vi "Generation.vi"(8 "error in":errorcluster, 10 "queue in":refnum<queue>, 11 "User Event in":refnum<user-event>) -> (0 "error out":errorcluster)   [LabVIEW 2016]
uses:
  DataEvent.ctl
  DataEvent/EventType.ctl
  Generation/GenerationAndAcquisitionEnum.ctl
  FGV/GetSetEnum.ctl
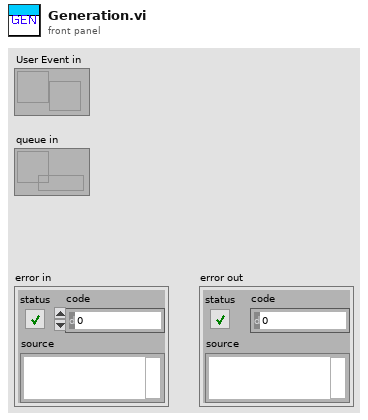
[diagram p1: front panel]
types:
  T1 = typedef "GenerationAndAcquisitionEnum.ctl" = enum16{"Idle", "Initialization", "GenerationAndPlayback", "End", "Error"}
  T2 = typedef "GetSetEnum.ctl" = enum16{"Init", "Get", "Set"}
  T3 = typedef "DataEvent.ctl" = cluster{"event type":T4, "data":variant}
  T4 = typedef "EventType.ctl" = enum16{"spectrum", "time", "exit"}
  T5 = typedef "ASIOData.ctl" = cluster{"Buffer Config":cluster{"# buffers":i32, "Buffer size":i32, "unit (ms)":enum16{"time (ms)", "Samples"}}, "Format (44kHz, 16Bit, stereo)":cluster{"Rate":i32, "Bits":i32, "Channels":u32}, "Play":bool, "Exit":bool}
  T6 = cluster{"# buffers":i32, "Buffer size":i32, "unit (ms)":enum16{"time (ms)", "Samples"}}
  T7 = typedef "SoundHandle.ctl" = cluster{"DeviceID":u16, "Samples/buf":u32, "Sampl rate":u32, "Bits/sample":u16, "Channels":u8, "Opened":bool}
  T8 = typedef "FMInfo.ctl" = cluster{"buffer size":i32, "bits":i32, "CarrierInfo":cluster{"frequency":dbl, "amplitude":dbl, "sample rate":i32, "waveform type":T9}, "ModulatorInfo":cluster{"frequency":dbl, "amplitude":dbl, "sample rate":i32, "waveform type":T9}, "Feedback":bool}
  T9 = typedef "WaveformType.ctl" = enum16{"Sine", "Triangle", "Square", "Sawtooth"}
  T10 = typedef "FilterInfo.ctl" = cluster{"filter type":T11, "high cutoff freq: fh":dbl, "low cutoff freq: fl":dbl, "order":i32}
  T11 = typedef "NI_AALBase.lvlib/Filter Passband Type.ctl" = enum32{"Lowpass", "Highpass", "Bandpass", "Bandstop"}
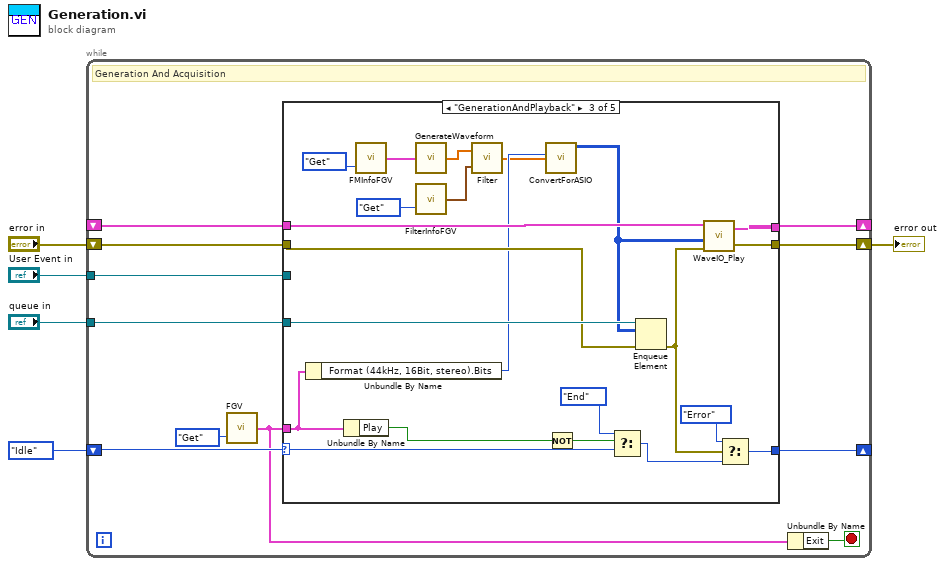
[diagram p0: block diagram]
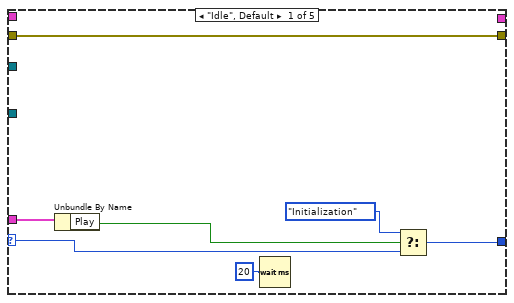
[diagram p2: hidden frame]
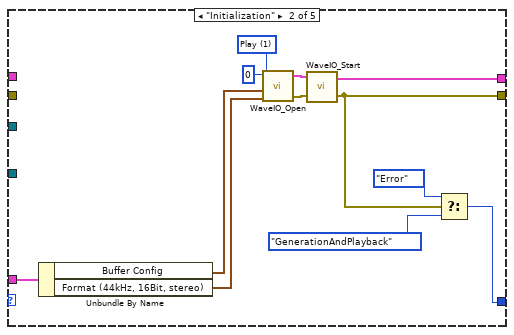
[diagram p3: hidden frame]
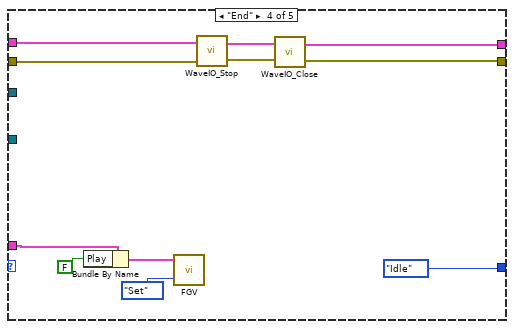
[diagram p4: hidden frame]
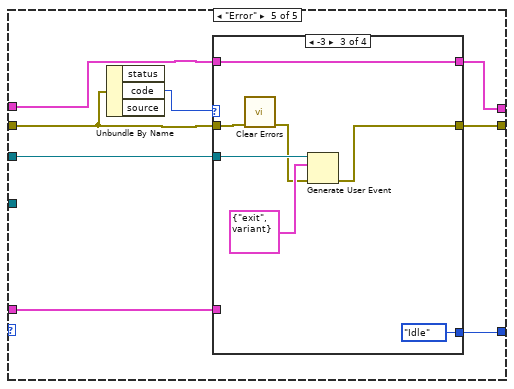
[diagram p5: hidden frame]
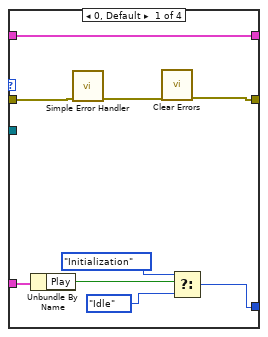
[diagram p6: hidden frame]
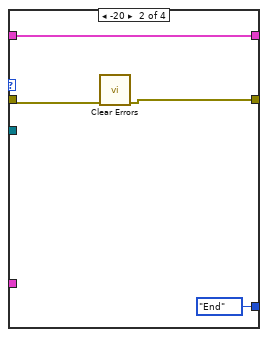
[diagram p7: hidden frame]
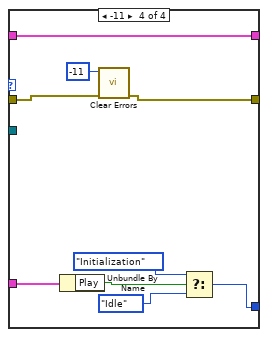
[diagram p8: hidden frame]
diagram:
  n1 = while {
    shift-right: [w9] -> _
    shift-left: GenerationAndAcquisitionEnum."Idle" -> [w10]
    shift-right: [w15] -> _
    shift-left: _ -> [w14]
    shift-right: [w12] -> w4
    shift-left: "error in" -> [w13]
    tunnel: "queue in" -> [w11]
    tunnel: "User Event in" -> [w6]
    stop <- w7 stop-if-true
    # "Generation And Acquisition"
    n2 = call "FGV.vi"("GetSetEnum"=GetSetEnum."Get") -> ("ASIODataOut"=w8:T5)  [unwired: 1 in]
    n3 = case shown="\"GenerationAndPlayback\"" w10 {
      selector: w10 -> [w23 _ w55 _ _]
      tunnel: [_ w32 w57 w66 w74] -> w15
      tunnel: [w20 w27 w53 w63 w76] -> w12
      tunnel: w14 -> [_ _ w56 w68 w75]
      tunnel: w13 -> [w20 _ w51 w65 w73]
      tunnel: w11 -> [_ _ w52 _ _]
      tunnel: [w18 w25 w43 GenerationAndAcquisitionEnum."Idle" w71] -> w9
      tunnel: w8 -> [w17 w24 w41 w59 w70]
      tunnel: w6 -> [_ _ _ _ w69]
      frame "Idle", Default {
        n4 = Unbundle By Name(w17) -> ("Play"=w19:bool)
        n5 = Wait (ms)(milliseconds to wait=u32 20) -> ()  [unwired: 1 out]
        n6 = Select(t=GenerationAndAcquisitionEnum."Initialization", s=w19, f=w23) -> (s? t:f=w18:T1)
      }
      frame "Initialization" {
        w34 = u16 1 items=["Record", "Play", "Loopback", "ASIO input", "ASIO output", "Record (WASAPI)", "Play (WASAPI)", "Record Combi", "Play Combi"] ("device type (Record)")
        n7 = Unbundle By Name(w24) -> ("Buffer Config"=w29:T6, "Format (44kHz, 16Bit, stereo)"=w28:cluster{"Rate":i32, "Bits":i32, "Channels":u32})
        n8 = call "WaveIO_Open.vi"("idev"=u32 0, "device type (Record)"=w34, "Buffer Config"=w29, "Format (44kHz, 16Bit, stereo)"=w28) -> ("Sound Handle Out"=w33:T7, "error out"=w31:errorcluster)  [unwired: 3 in]
        n9 = call "WaveIO_Start.vi"("error in (no error)"=w31, "Handle"=w33) -> ("error out"=w27:errorcluster, "Handle Out"=w32:T7)
        n10 = Select(t=GenerationAndAcquisitionEnum."Error", s=w27, f=GenerationAndAcquisitionEnum."GenerationAndPlayback") -> (s? t:f=w25:T1)
      }
      frame "GenerationAndPlayback" {
        n11 = Unbundle By Name(w41) -> ("Format (44kHz, 16Bit, stereo).Bits"=w40:i32)
        n12 = Unbundle By Name(w41) -> ("Play"=w46:bool)
        n13 = call "FMInfoFGV.vi"("GetSetEnum"=GetSetEnum."Get") -> ("FMInfoOut"=w45:T8)  [unwired: 1 in]
        n14 = call "GenerateWaveform.vi"("FMInfo"=w45) -> ("generated signal"=w39:dbl[])
        n15 = call "FilterInfoFGV.vi"("GetSet enum"=GetSetEnum."Get") -> ("FilterInfo out"=w36:T10)  [unwired: 1 in]
        n16 = call "Filter.vi"("filter info"=w36, "signal to filter"=w39) -> ("filtered signal"=w38:dbl[])
        n17 = call "ConvertForASIO.vi"("bits"=w40, "input channel"=w38) -> ("signal for ASIO"=w42:i32[][])  [unwired: 9 in]
        n18 = Not(x=w46) -> (.not. x?=w50:bool)
        n19 = Select(t=GenerationAndAcquisitionEnum."End", s=w50, f=w55) -> (s? t:f=w48:T1)
        n20 = Enqueue Element(queue=w52, element=w42, error in (no error)=w51) -> (error out=w49:errorcluster)  [unwired: 1 in, 2 out]
        n21 = call "WaveIO_Play.vi"("error in (no error)"=w49, "data"=w42, "Handle"=w56) -> ("error out"=w53:errorcluster, "Handle Out"=w57:T7)  [unwired: 1 in]
        n22 = Select(t=GenerationAndAcquisitionEnum."Error", s=w49, f=w48) -> (s? t:f=w43:T1)
      }
      frame "End" {
        n23 = Bundle By Name(cluster=w59, "Play"=FALSE) -> (w58:T5)
        n24 = call "FGV.vi"("GetSetEnum"=GetSetEnum."Set", "ASIODataIn"=w58) -> ()  [unwired: 1 out]
        n25 = call "WaveIO_Stop.vi"("error in (no error)"=w65, "Handle"=w68) -> ("error out"=w64:errorcluster, "Handle Out"=w67:T7)
        n26 = call "WaveIO_Close.vi"("error in (no error)"=w64, "Handle"=w67) -> ("error out"=w63:errorcluster, "Handle Out"=w66:T7)
      }
      frame "Error" {
        n27 = Unbundle By Name(w73) -> ("code"=w72:i32)  [unwired: 2 out]
        n28 = case shown="-3" w72 {
          tunnel: w73 -> [w83 w89 w91 w105]
          tunnel: [w85 w88 w92 w104] -> w76
          tunnel: w75 -> [w84 w86 w96 w103]
          tunnel: [w84 w86 w96 w103] -> w74
          tunnel: [w80 GenerationAndAcquisitionEnum."End" GenerationAndAcquisitionEnum."Idle" w99] -> w71
          tunnel: w70 -> [w78 _ _ w98]
          tunnel: w69 -> [_ _ w94 _]
          frame 0, Default {
            n29 = Unbundle By Name(w78) -> ("Play"=w77:bool)
            n30 = call <vilib>:"Simple Error Handler.vi"("error in (no error)"=w83) -> ("error out"=w82:errorcluster)  [unwired: 4 in, 4 out]
            n31 = call <vilib>:"Clear Errors.vi"("error in (no error)"=w82) -> ("error out"=w85:errorcluster)  [unwired: 5 in, 1 out]
            n32 = Select(t=GenerationAndAcquisitionEnum."Initialization", s=w77, f=GenerationAndAcquisitionEnum."Idle") -> (s? t:f=w80:T1)
          }
          frame -20 {
            n33 = call <vilib>:"Clear Errors.vi"("error in (no error)"=w89) -> ("error out"=w88:errorcluster)  [unwired: 5 in, 1 out]
          }
          frame -3 {
            n34 = call <vilib>:"Clear Errors.vi"("error in (no error)"=w91) -> ("error out"=w90:errorcluster)  [unwired: 5 in, 1 out]
            n35 = Generate User Event(user event=w94, event data cluster=T3 {"event type"=enum."exit", "data"=variant} ("event data"), error in=w90) -> (error out=w92:errorcluster)  [unwired: 1 in, 1 out]
          }
          frame -11 {
            n36 = Unbundle By Name(w98) -> ("Play"=w97:bool)
            n37 = call <vilib>:"Clear Errors.vi"("error in (no error)"=w105, "specific error code to clear (0: all)"=-11) -> ("error out"=w104:errorcluster)  [unwired: 4 in, 1 out]
            n38 = Select(t=GenerationAndAcquisitionEnum."Initialization", s=w97, f=GenerationAndAcquisitionEnum."Idle") -> (s? t:f=w99:T1)
          }
        }
      }
    }
    n39 = Unbundle By Name(w8) -> ("Exit"=w7:bool)
  }
  "error out" <- w4
